vi "OceanOpticsRecordSpectra.vi"(1 "Boxcar Width":i32, 2 "Scans to Average":i32, 3 "EDC Enable":i32, 4 "NLC Enable":i32, 5 "error in (no error)":errorcluster, 6 "lampOn":i32, 7 "N Integrations":i32, 8 "Int. Time (microsec)":i32, 9 "lampOn 2":i32, 10 "Spectrometer Index":i32, 11 "enable":i16) -> (12 "getName":string, 14 "getSerialNumber":string, 15 "XY Graph":cluster{"Y":dbl[], "Y":dbl[]}[](array[cluster]), 16 "Array":dbl[][](array[numeric]), 19 "error out":errorcluster)   [LabVIEW 2023]
uses:
  C:/Program Files/Ocean Optics/OmniDriver/OOI_HOME/NETOmniDriver-NET40.dll
  Program Files/Ocean Optics/OmniDriver/OOI_HOME/NETOmniDriver-NET40.dll
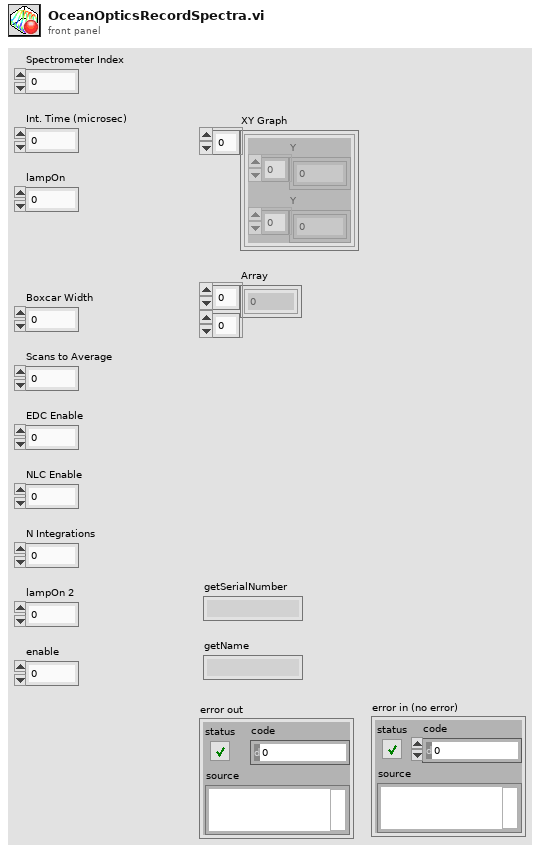
[diagram p1: front panel]
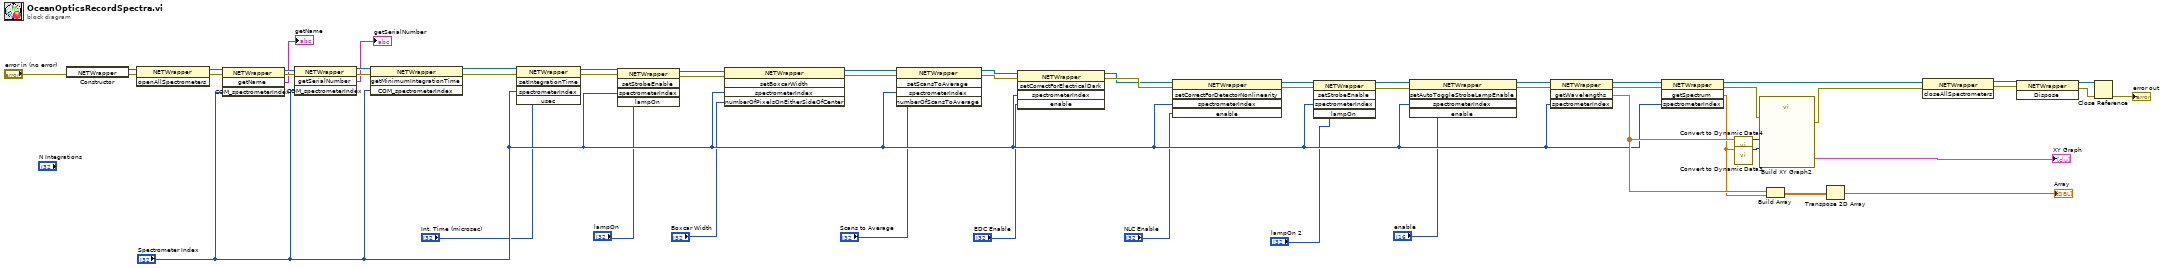
[diagram p0: block diagram]
diagram:
  n1 = constructor class="NETWrapper"(error in="error in (no error)") -> (reference out=w54:refnum<k24>, error out=w55:errorcluster)  [unwired: 2 in, 1 out]
  n2 = invoke class="NETWrapper" method="openAllSpectrometers"(reference=w54, error in=w55) -> (reference out=w48:refnum<k24>, error out=w49:errorcluster)  [unwired: 1 in, 1 out]
  n3 = invoke class="NETWrapper" method="getName"(reference=w48, error in=w49, "COM_spectrometerIndex"="Spectrometer Index") -> (reference out=w50:refnum<k24>, error out=w51:errorcluster, "getName"=→"getName":string)  [unwired: 1 in, 1 out]
  n4 = invoke class="NETWrapper" method="getSerialNumber"(reference=w50, error in=w51, "COM_spectrometerIndex"="Spectrometer Index") -> (reference out=w52:refnum<k24>, error out=w53:errorcluster, "getSerialNumber"=→"getSerialNumber":string)  [unwired: 1 in, 1 out]
  n5 = invoke class="NETWrapper" method="getMinimumIntegrationTime"(reference=w52, error in=w53, "COM_spectrometerIndex"="Spectrometer Index") -> (reference out=w10:refnum<k24>, error out=w9:errorcluster)  [unwired: 1 in, 2 out]
  n6 = invoke class="NETWrapper" method="setIntegrationTime"(reference=w10, error in=w9, "spectrometerIndex"="Spectrometer Index", "usec"="Int. Time (microsec)") -> (reference out=w26:refnum<k24>, error out=w27:errorcluster)  [unwired: 1 in, 3 out]
  n7 = invoke class="NETWrapper" method="setStrobeEnable"(reference=w26, error in=w27, "spectrometerIndex"="Spectrometer Index", "lampOn"="lampOn") -> (reference out=w28:refnum<k24>, error out=w29:errorcluster)  [unwired: 1 in, 3 out]
  n8 = invoke class="NETWrapper" method="setBoxcarWidth"(reference=w28, error in=w29, "spectrometerIndex"="Spectrometer Index", "numberOfPixelsOnEitherSideOfCenter"="Boxcar Width") -> (reference out=w20:refnum<k24>, error out=w21:errorcluster)  [unwired: 1 in, 3 out]
  n9 = invoke class="NETWrapper" method="setScansToAverage"(reference=w20, error in=w21, "spectrometerIndex"="Spectrometer Index", "numberOfScansToAverage"="Scans to Average") -> (reference out=w22:refnum<k24>, error out=w24:errorcluster)  [unwired: 1 in, 3 out]
  n10 = invoke class="NETWrapper" method="setCorrectForElectricalDark"(reference=w22, error in=w24, "spectrometerIndex"="Spectrometer Index", "enable"="EDC Enable") -> (reference out=w23:refnum<k24>, error out=w25:errorcluster)  [unwired: 1 in, 3 out]
  n11 = invoke class="NETWrapper" method="setCorrectForDetectorNonlinearity"(reference=w23, error in=w25, "spectrometerIndex"="Spectrometer Index", "enable"="NLC Enable") -> (reference out=w30:refnum<k24>, error out=w31:errorcluster)  [unwired: 1 in, 3 out]
  n12 = invoke class="NETWrapper" method="setStrobeEnable"(reference=w30, error in=w31, "spectrometerIndex"="Spectrometer Index", "lampOn"="lampOn 2") -> (reference out=w32:refnum<k24>, error out=w33:errorcluster)  [unwired: 1 in, 3 out]
  n13 = invoke class="NETWrapper" method="setAutoToggleStrobeLampEnable"(reference=w32, error in=w33, "spectrometerIndex"="Spectrometer Index", "enable"="enable") -> (reference out=w34:refnum<k24>, error out=w35:errorcluster)  [unwired: 1 in, 3 out]
  n14 = invoke class="NETWrapper" method="getWavelengths"(reference=w34, error in=w35, "spectrometerIndex"="Spectrometer Index") -> (reference out=w16:refnum<k24>, error out=w17:errorcluster, "getWavelengths"=w38:dbl[])  [unwired: 1 in, 1 out]
  n15 = invoke class="NETWrapper" method="getSpectrum"(reference=w16, error in=w17, "spectrometerIndex"="Spectrometer Index") -> (reference out=w15:refnum<k24>, error out=w36:errorcluster, "getSpectrum"=w37:dbl[])  [unwired: 1 in, 1 out]
  n16 = call "Convert to Dynamic Data4"("Array"=w38) -> ("Dynamic Data Type"=w18:dynamicdata)  [unwired: 3 out]
  n17 = call "Convert to Dynamic Data3"("Array"=w37) -> ("Dynamic Data Type"=w19:dynamicdata)  [unwired: 3 out]
  n18 = call "Build XY Graph2"("error in (no error)"=w36, "Y Input"=w19, "X Input"=w18) -> ("error out"=w14:errorcluster, "XY Graph"=→"XY Graph":cluster{"Y":dbl[], "Y":dbl[]}[])  [unwired: 2 in, 5 out]
  n19 = Build Array(w38, w37) -> (w39:dbl[][])
  n20 = Transpose 2D Array(2D array=w39) -> (transposed array=→"Array":dbl[][])
  n21 = invoke class="NETWrapper" method="closeAllSpectrometers"(reference=w15, error in=w14) -> (reference out=w41:refnum<k24>, error out=w42:errorcluster)  [unwired: 1 in, 1 out]
  n22 = invoke class="NETWrapper" method="Dispose"(reference=w41, error in=w42) -> (reference out=w43:refnum<k24>, error out=w44:errorcluster)  [unwired: 1 in, 1 out]
  n23 = Close Reference(reference=w43, error in (no error)=w44) -> (error out=→"error out":errorcluster)
